vi "setCurrentSortSearch.vi"(8 "error in (no error)":errorcluster, 10 "CurrentSortSearch":dbl, 11 "BasicSortedList in":refnum<class "BasicSortedList.lvclass">) -> (0 "error out":errorcluster, 3 "BasicSortedList out":refnum<class "BasicSortedList.lvclass">)   [LabVIEW 2009, in "BasicSortedList.lvclass"]
doc: "Sets the current value you are searching for in the sorted list."
uses:
  BasicSortedList.lvclass
  BasicSortedList.lvclass/BasicSortedList.ctl
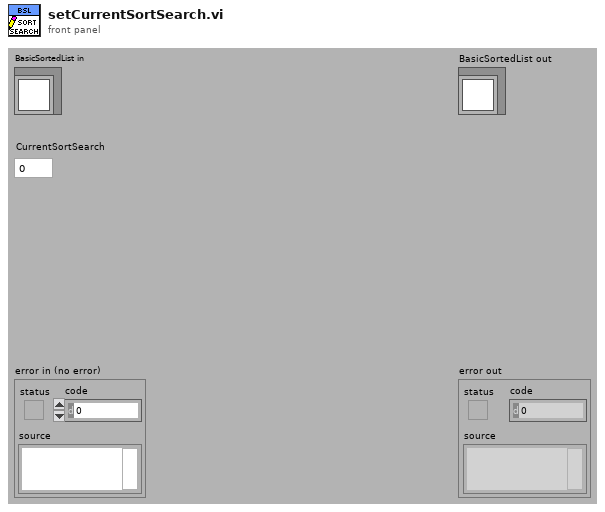
[diagram p1: front panel]
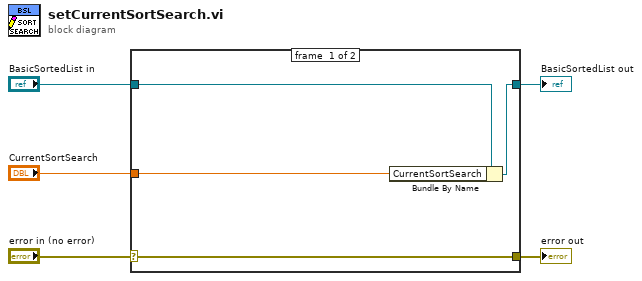
[diagram p0: block diagram]
diagram:
  n1 = case shown="No Error" "error in (no error)" {
    selector: "error in (no error)" -> [w9 w10]
    tunnel: [w9 w10] -> w4
    tunnel: [w7 w11] -> w2
    tunnel: "BasicSortedList in" -> [w8 w11]
    tunnel: "CurrentSortSearch" -> [w6 _]
    frame #0 {
      n2 = Bundle By Name(cluster=w8, "CurrentSortSearch"=w6) -> (w7:refnum<class "BasicSortedList.lvclass">)
    }
    frame #1 {
    }
  }
  "error out" <- w4
  "BasicSortedList out" <- w2
